vi "PWM no errors.vi"() -> ()   [LabVIEW 2018]
uses:
  <vilib>/DAQmx/create/channels.llb/DAQmx Create Channel (CO-Pulse Generation-Frequency).vi
  <vilib>/DAQmx/configure/timing.llb/DAQmx Timing (Implicit).vi
  <resource>/objmgr/daqmx.rc
panel:
  in  "CO.Pulse.DutyCyc":dbl
  in  "Stop":bool caption="stop"
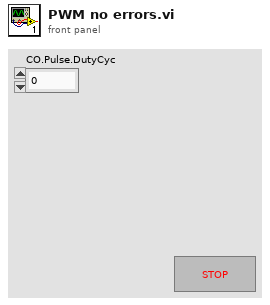
[diagram p1: front panel]
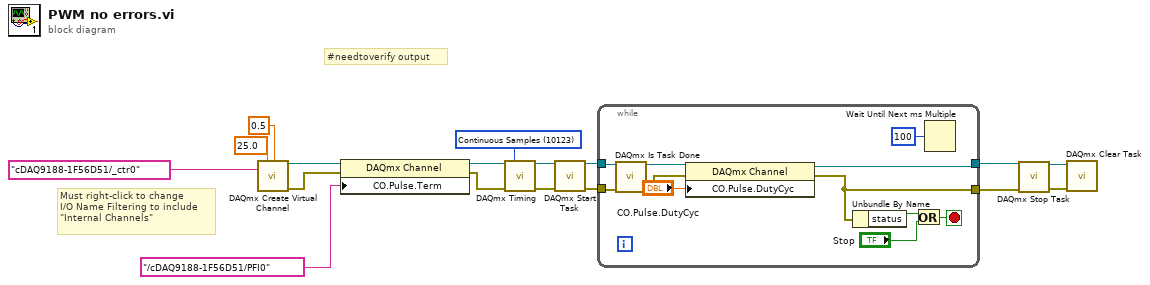
[diagram p0: block diagram]
diagram:
  w13 = 10123 items=["Finite Samples"=10178, "Continuous Samples"=10123] ("sample mode")
  # "#needtoverify output"
  # "Must right-click to change\nI/O Name Filtering to include\n\"Internal Channels\""
  n1 = call-poly <vilib>:"DAQmx Create Virtual Channel.vi"("frequency"=25.0 ("Frequency"), "duty cycle"=0.5 ("Duty Cycle"), "counter"=tag "cDAQ9188-1F56D51/_ctr0" ("Counter(s)")) -> ("task out"=w9:refnum<k21>, "error out"=w8:errorcluster)  [unwired: 11 in]
  n2 = property class="DAQmx Channel"(reference=w9, error in=w8, "CO.Pulse.Term"=tag "/cDAQ9188-1F56D51/PFI0") -> (reference out=w6:refnum<k21>, error out=w7:errorcluster)
  n3 = call-poly <vilib>:"DAQmx Timing.vi"("task/channels in"=w6, "sample mode"=w13, "error in"=w7) -> ("task out"=w14:refnum<k21>, "error out"=w15:errorcluster)  [unwired: 11 in]
  n4 = call <vilib>:"DAQmx Start Task.vi"("task/channels in"=w14, "error in"=w15) -> ("task out"=w16:refnum<k21>, "error out"=w17:errorcluster)  [unwired: 12 in]
  n5 = while {
    tunnel: w17 -> [w27]
    tunnel: w16 -> [w28]
    tunnel: [w20] -> w3
    tunnel: [w19] -> w4
    stop <- w25 stop-if-true
    n6 = call <vilib>:"DAQmx Is Task Done.vi"("task/channels in"=w28, "error in"=w27) -> ("task out"=w22:refnum<k21>, "error out"=w21:errorcluster)  [unwired: 11 in, 1 out]
    n7 = property class="DAQmx Channel"(reference=w22, error in=w21, "CO.Pulse.DutyCyc"="CO.Pulse.DutyCyc") -> (reference out=w20:refnum<k21>, error out=w19:errorcluster)
    n8 = Unbundle By Name(w19) -> ("status"=w24:bool)
    n9 = Or(x=w24, y="Stop") -> (x .or. y?=w25:bool)
    n10 = Wait Until Next ms Multiple(millisecond multiple=u32 100) -> ()  [unwired: 1 out]
  }
  n11 = call <vilib>:"DAQmx Stop Task.vi"("task/channels in"=w3, "error in"=w4) -> ("task out"=w2:refnum<k21>, "error out"=w1:errorcluster)  [unwired: 12 in]
  n12 = call <vilib>:"DAQmx Clear Task.vi"("task in"=w2, "error in"=w1) -> ()  [unwired: 13 in, 1 out]
